vi "test Get Parameters.vi"(8 "error in":errorcluster, 11 "TestCase in":refnum<class "Scripting.lvclass">) -> (0 "error out":errorcluster, 3 "TestCase out":refnum<class "Scripting.lvclass">)   [LabVIEW 2020, in "Scripting.lvclass"]
uses:
  Scripting.lvclass
  Shared/Parameter Definition.ctl
  Encoding and Decoding/Encoding.ctl
  Shared/Label Properties.ctl
  Scripting.lvclass/Scripting.ctl
  Scripting/Constants.vi
  <vilib>/NI VeriStand/Custom Device Tools/Custom Device Utility Library/NI VeriStand - Search for Item by GUID.vi
  <vilib>/addons/_JKI Toolkits/VI Tester/TestCase.llb/TestCase.lvclass
  Scripting/Ballard ARINC 429 Scripting.lvlib
  Encoding and Decoding/Encoding and Decoding.lvlib
  <vilib>/NI VeriStand/Custom Device Tools/Custom Device Utility Library/Custom Device Utility Library.lvlib
  <vilib>/NI VeriStand/Custom Device API/Custom Device API.lvlib
  C:/Program Files (x86)/National Instruments/LabVIEW 2020/vi.lib/addons/_JKI Toolkits/VI Tester/TestCase.llb/TestCase.lvclass
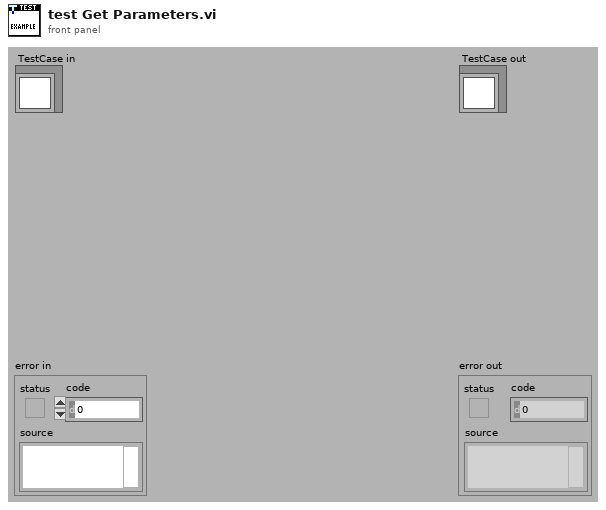
[diagram p1: front panel]
types:
  T1 = typedef "Label Properties.ctl" = cluster{"label (Dec)":i32, "SDI value":u8, "SDI enabled":bool}
  T2 = typedef "Parameter Definition.ctl" = cluster{"start index":i32, "size":i32, "encoding":T3, "signed":bool, "scale multiplier":dbl, "scale offset":dbl}
  T3 = typedef "Encoding and Decoding.lvlib/Encoding.ctl" = enum16{"BNR", "BCD", "Discrete"}
  T4 = typedef "Custom Device API.lvlib/Custom Device Item Ref.ctl" = u64
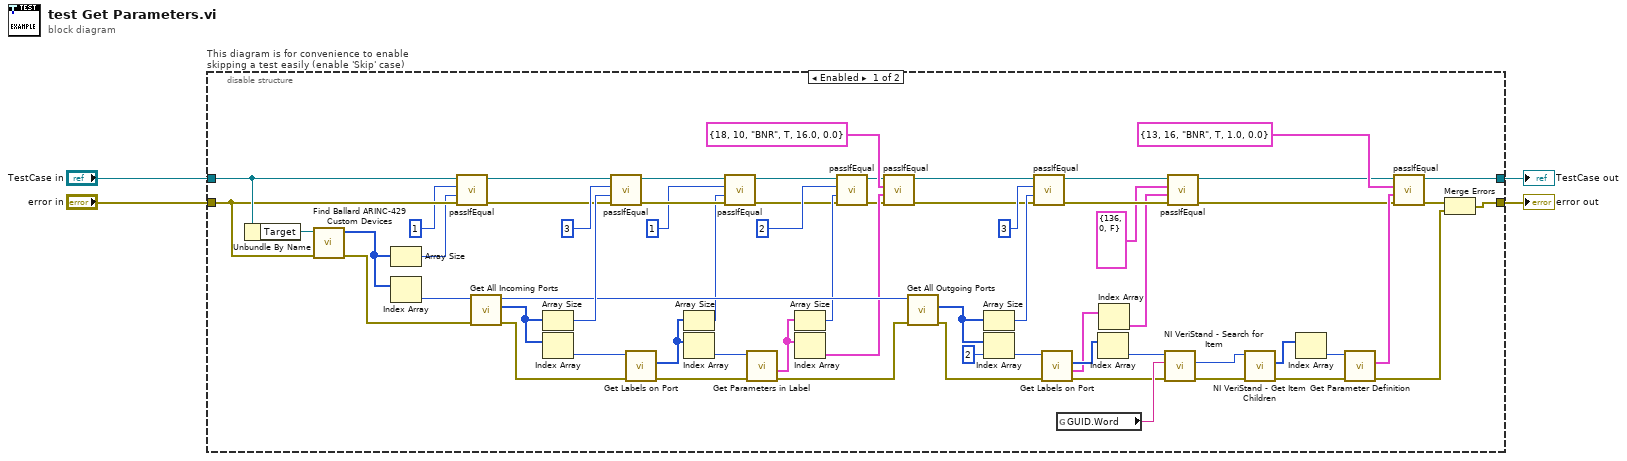
[diagram p0: block diagram]
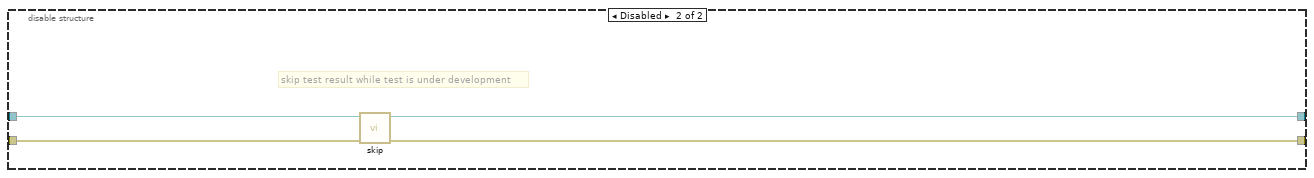
[diagram p2: hidden frame]
diagram:
  n1 = disable-structure "This diagram is for convenience to enable skipping a test easily (enable 'Skip' case)" shown="Enabled" {
    disable-tunnel: "TestCase in" -> [w64 w71]
    disable-tunnel: [w43 w69] -> w1
    disable-tunnel: [w45 w70] -> w3
    disable-tunnel: "error in" -> [w63 w68]
    frame Enabled {
      n2 = Unbundle By Name(w64) -> ("Target"=w66:refnum<k24>)
      n3 = call "Find Ballard ARINC-429 Custom Devices.vi"("error in"=w63, "target"=w66) -> ("error out"=w54:errorcluster, "Ballard ARINC-429 custom devices"=w62:u64[])  [unwired: 8 in]
      n4 = Array Size(array=w62) -> (size(s)=w60:i32)
      n5 = Index Array(array=w62) -> (element=w65:u64)  [unwired: 1 in]
      n6 = call-dynamic "passIfEqual.vi"("error in (no error)"=w63, "y"=w60, "x"=1 ("size(s)"), "TestCase in"=w64) -> ("error out"=w55:errorcluster, "TestCase out"=w56:refnum<class "Scripting.lvclass">)  [unwired: 6 in]
      n7 = call "Get All Incoming Ports.vi"("error in"=w54, "Ballard ARINC 429 ref"=w65) -> ("error out"=w24:errorcluster, "Port refs"=w59:T4[], "Ballard ARINC 429 ref out"=w53:T4)  [unwired: 7 in]
      n8 = Array Size(array=w59) -> (size(s)=w57:i32)
      n9 = Index Array(array=w59) -> (element=w26:T4)  [unwired: 1 in]
      n10 = call-dynamic "passIfEqual.vi"("error in (no error)"=w55, "y"=w57, "x"=3 ("size(s)"), "TestCase in"=w56) -> ("error out"=w37:errorcluster, "TestCase out"=w38:refnum<class "Scripting.lvclass">)  [unwired: 6 in]
      n11 = call "Get Labels on Port.vi"("error in"=w24, "port ref"=w26) -> ("error out"=w23:errorcluster, "label references"=w25:T4[])  [unwired: 6 in, 2 out]
      n12 = Array Size(array=w25) -> (size(s)=w34:i32)
      n13 = Index Array(array=w25) -> (element=w36:T4)  [unwired: 1 in]
      n14 = call-dynamic "passIfEqual.vi"("error in (no error)"=w37, "y"=w34, "x"=1 ("size(s)"), "TestCase in"=w38) -> ("error out"=w29:errorcluster, "TestCase out"=w30:refnum<class "Scripting.lvclass">)  [unwired: 6 in]
      n15 = call "Get Parameters in Label.vi"("error in"=w23, "label ref"=w36) -> ("error out"=w40:errorcluster, "parameter definitions"=w33:T2[])  [unwired: 6 in, 2 out]
      n16 = Array Size(array=w33) -> (size(s)=w31:i32)
      n17 = Index Array(array=w33) -> (element=w39:T2)  [unwired: 1 in]
      n18 = call-dynamic "passIfEqual.vi"("error in (no error)"=w29, "y"=w31, "x"=2 ("size(s)"), "TestCase in"=w30) -> ("error out"=w27:errorcluster, "TestCase out"=w28:refnum<class "Scripting.lvclass">)  [unwired: 6 in]
      n19 = call-dynamic "passIfEqual.vi"("error in (no error)"=w27, "y"=w39, "x"=T2 {"start index"=18, "size"=10, "encoding"=enum."BNR", "signed"=TRUE, "scale multiplier"=16.0, "scale offset"=0.0} ("parameter definition"), "TestCase in"=w28) -> ("error out"=w49:errorcluster, "TestCase out"=w50:refnum<class "Scripting.lvclass">)  [unwired: 6 in]
      n20 = call "Get All Outgoing Ports.vi"("error in"=w40, "Ballard ARINC 429 ref"=w53) -> ("error out"=w22:errorcluster, "Port refs"=w48:T4[])  [unwired: 7 in, 1 out]
      n21 = Array Size(array=w48) -> (size(s)=w51:i32)
      n22 = Index Array(array=w48, index=2) -> (element=w21:T4)
      n23 = call-dynamic "passIfEqual.vi"("error in (no error)"=w49, "y"=w51, "x"=3 ("size(s)"), "TestCase in"=w50) -> ("error out"=w15:errorcluster, "TestCase out"=w16:refnum<class "Scripting.lvclass">)  [unwired: 6 in]
      n24 = call "Get Labels on Port.vi"("error in"=w22, "port ref"=w21) -> ("error out"=w17:errorcluster, "labels properties"=w12:T1[], "label references"=w20:T4[])  [unwired: 6 in, 1 out]
      n25 = global read "Constants.vi" "GUID.Word"() -> (w18:string)
      n26 = Index Array(array=w20) -> (element=w19:T4)  [unwired: 1 in]
      n27 = Index Array(array=w12) -> (element=w11:T1)  [unwired: 1 in]
      n28 = call-poly <vilib>:"NI VeriStand - Search for Item.vi"("error in"=w17, "Item GUID"=w18, "Section Ref in"=w19) -> ("error out"=w8:errorcluster, "Item Ref"=w9:T4)  [unwired: 5 in, 2 out]
      n29 = call-dynamic "passIfEqual.vi"("error in (no error)"=w15, "y"=w11, "x"=T1 {"label (Dec)"=136, "SDI value"=0, "SDI enabled"=FALSE} ("element"), "TestCase in"=w16) -> ("error out"=w13:errorcluster, "TestCase out"=w14:refnum<class "Scripting.lvclass">)  [unwired: 6 in]
      n30 = call <vilib>:"NI VeriStand - Get Item Children.vi"("error in (no error)"=w8, "Item Ref in"=w9) -> ("error out"=w7:errorcluster, "Child Refs"=w5:T4[])  [unwired: 6 in, 2 out]
      n31 = Index Array(array=w5) -> (element=w6:T4)  [unwired: 1 in]
      n32 = call "Get Parameter Definition.vi"("error in"=w7, "parameter ref in"=w6) -> ("error out"=w46:errorcluster, "parameter definition"=w44:T2)  [unwired: 7 in, 1 out]
      n33 = call-dynamic "passIfEqual.vi"("error in (no error)"=w13, "y"=w44, "x"=T2 {"start index"=13, "size"=16, "encoding"=enum."BNR", "signed"=TRUE, "scale multiplier"=1.0, "scale offset"=0.0} ("parameter definition"), "TestCase in"=w14) -> ("error out"=w42:errorcluster, "TestCase out"=w43:refnum<class "Scripting.lvclass">)  [unwired: 6 in]
      n34 = Merge Errors(w42, w46) -> (w45:errorcluster)
    }
    frame Disabled {
      # "skip test result while test is under development"
      n35 = call <vilib>:"skip.vi"("error in (no error)"=w68, "TestCase in"=w71) -> ("error out"=w70:errorcluster, "TestCase out"=w69:refnum<class "Scripting.lvclass">)  [unwired: 8 in]
    }
  }
  "error out" <- w3
  "TestCase out" <- w1
